vi "USRP_singlecarrierTDMUSRP1_withoutemu.vi"() -> ()   [LabVIEW 2021]
uses:
  <vilib>/addons/Modulation/Analog/controls/Complex Data Waveform.ctl
  <vilib>/Analysis/coordinate.llb/Angle Units.ctl
  <vilib>/Analysis/coordinate.llb/Angle Range (Degree).ctl
  <vilib>/Analysis/coordinate.llb/Wrap Angle (scalar).vi
  system stop.vi
  <vilib>/measure/matone.llb/Extract Single Tone Information 1 Chan (CDB).vi
  <instrlib>/niUSRP/niUSRP Fetch Rx Data (CDB Cluster).vi
  <instrlib>/niUSRP/niUSRP Write Tx Data (CDB Cluster).vi
  <vilib>/addons/Modulation/niAMT.lvlib
  <vilib>/measure/NI_MAPro.lvlib
  <vilib>/Analysis/NI_AAL_Angle.lvlib
panel:
  in  "Tab Control":T1(tab)
  in  "IQ rate Tx":dbl=400000.0 format="%#_6p"
  in  "Tx Gain":dbl format="%#_6f"
  in  "Tx IP":refnum<k15>="192.168.10.2"
  out "coerced IQ rate Tx":dbl=100000.0 format="%#_6p"
  out "coerced carrier frequency Tx":dbl=100000.0 format="%#_6p"
  in  "Rx IP":refnum<k15>="192.168.10.2"
  in  "Rx gain":dbl format="%#_6f"
  in  "Frequency":dbl=10000.0 format="%#_13g"
  in  "Duration":dbl=0.01 format="%#_13g"
  out "coerced IQ rate Rx":dbl=100000.0 format="%#_6p"
  out "coerced carrier frequency Rx":dbl=100000.0 format="%#_6p"
  in  "number of samples":i64=4000
  in  "carrier frequency":dbl=2400000000.0 format="%#_6p"
  in  "Phase in deg":dbl
  out "Waveform Graph":dbl[](graph)
  out "Boolean":bool
  out "detected frequency":dbl format="%.2p"
  out "detected Amplitude in dBm":dbl format="%.2p"
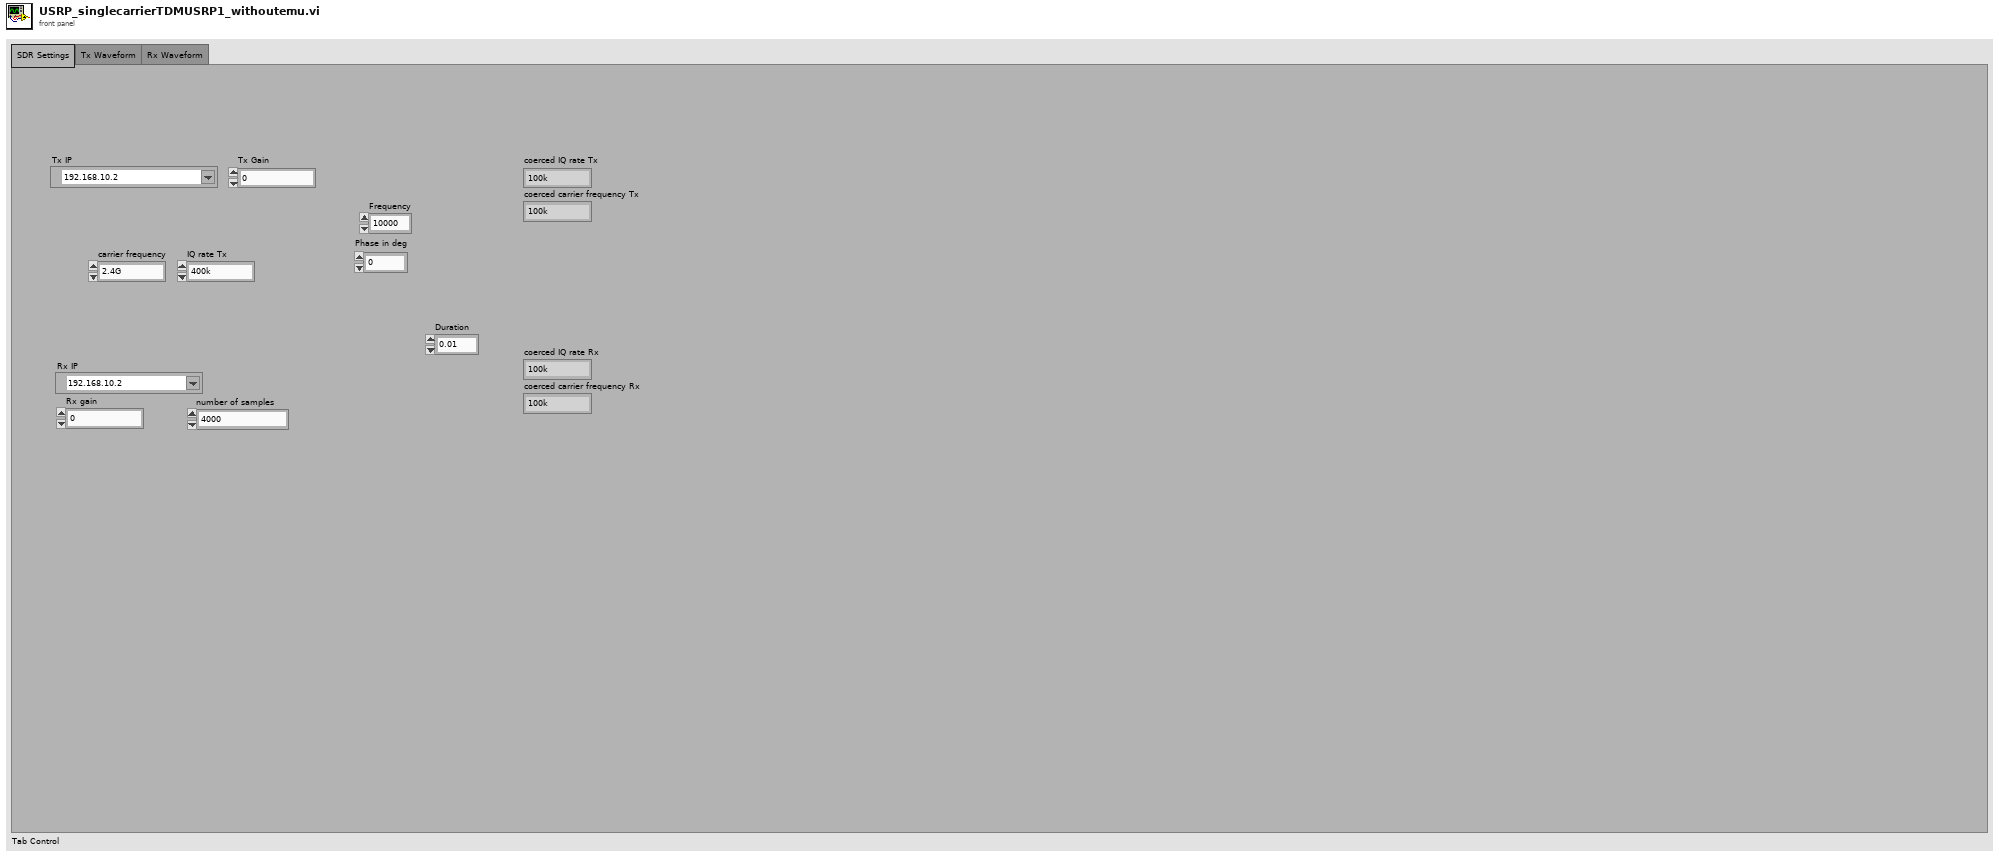
[diagram p1: front panel]
types:
  T1 = enum32{"SDR Settings", "Tx Waveform", "Rx Waveform"}
  T2 = typedef "niAMT.lvlib/Complex Data Waveform.ctl" = cluster{"t0":dbl, "dt":dbl, "Y":cdb[]}
  T3 = typedef "NI_AAL_Angle.lvlib/Angle Range (Degree).ctl" = u16
  T4 = typedef "NI_AAL_Angle.lvlib/Angle Units.ctl" = i32
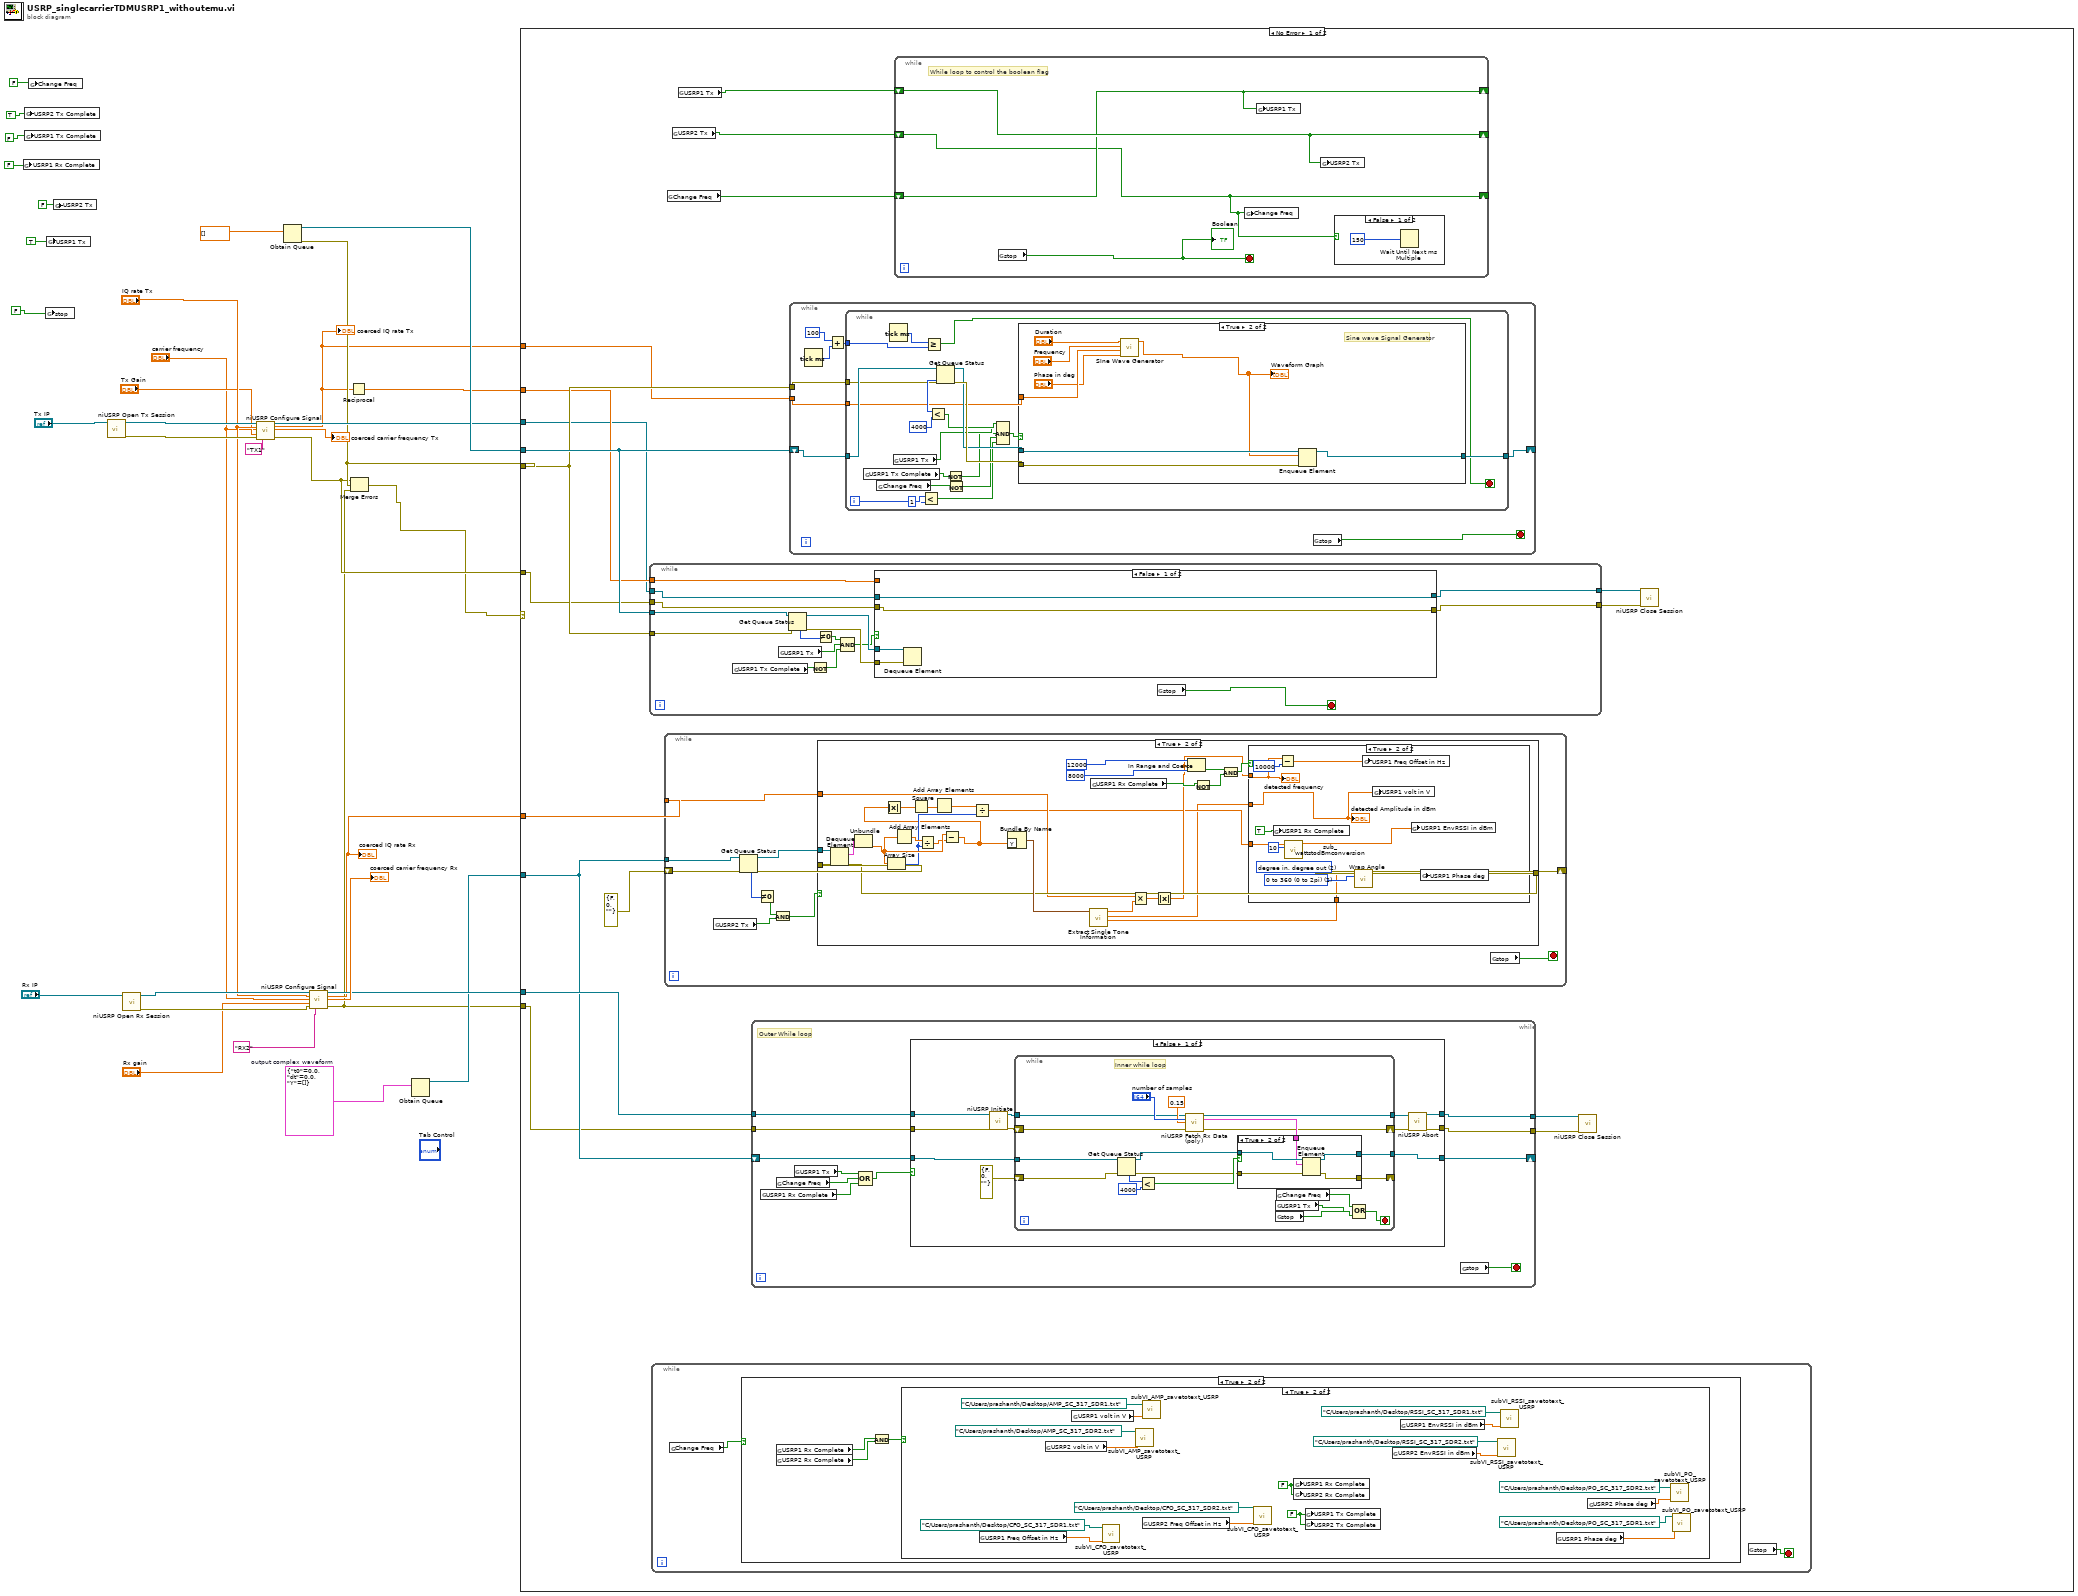
[diagram p0: block diagram]
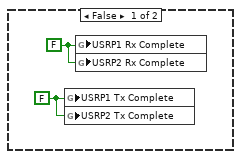
[diagram p3: hidden frame]
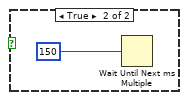
[diagram p4: hidden frame]
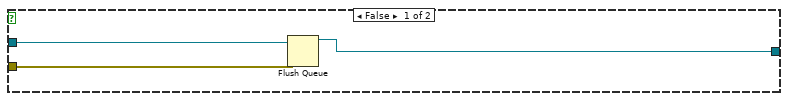
[diagram p5: hidden frame]
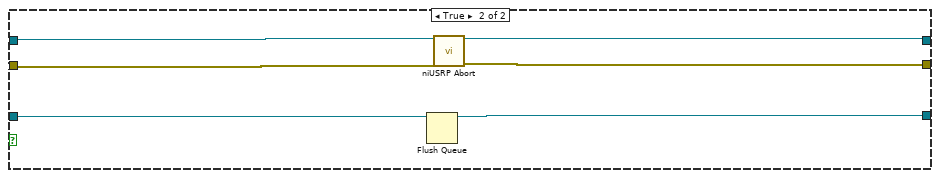
[diagram p7: hidden frame]
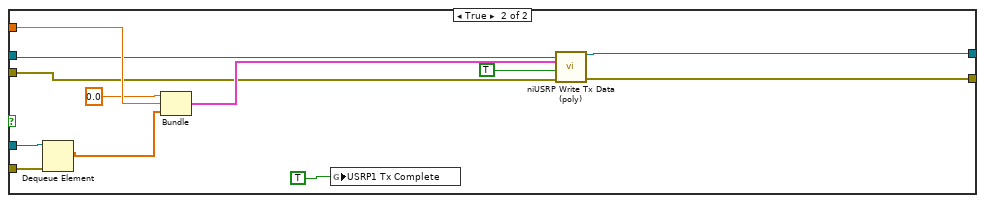
[diagram p10: hidden frame]
diagram:
  w8 = T2 {"t0"=0.0, "dt"=0.0, "Y"=[]}  # output complex waveform
  n1 = global write "system stop.vi" "USRP1 Rx Complete"(FALSE) -> ()
  n2 = global write "system stop.vi" "USRP2 Tx Complete"(TRUE) -> ()
  n3 = global write "system stop.vi" "USRP1 Tx Complete"(FALSE) -> ()
  n4 = global write "system stop.vi" "Change Freq"(FALSE) -> ()
  n5 = global write "system stop.vi" "stop"(FALSE) -> ()
  n6 = global write "system stop.vi" "USRP1 Tx"(TRUE) -> ()
  n7 = global write "system stop.vi" "USRP2 Tx"(FALSE) -> ()
  n8 = call <instrlib>:"niUSRP Open Tx Session.vi"("device names"="Tx IP") -> ("session handle out"=w33:refnum<k15>, "error out"=w32:errorcluster)  [unwired: 13 in]
  n9 = call <instrlib>:"niUSRP Open Rx Session.vi"("device names"="Rx IP") -> ("session handle out"=w30:refnum<k15>, "error out"=w29:errorcluster)  [unwired: 13 in]
  n10 = call <instrlib>:"niUSRP Configure Signal.vi"("session handle"=w33, "IQ rate"="IQ rate Tx", "carrier frequency"="carrier frequency", "gain"="Tx Gain", "error in (no error)"=w32, "active antenna"="TX1") -> ("session handle out"=w15:refnum<k15>, "coerced IQ rate"=w12:dbl, "coerced carrier frequency"=→"coerced carrier frequency Tx":dbl, "error out"=w11:errorcluster)  [unwired: 5 in, 1 out]
  "coerced IQ rate Tx" <- w12
  n11 = Obtain Queue(element data type=dbl[] []) -> (queue out=w16:refnum<queue>, error out=w13:errorcluster)  [unwired: 4 in, 1 out]
  n12 = call <instrlib>:"niUSRP Configure Signal.vi"("session handle"=w30, "IQ rate"="IQ rate Tx", "carrier frequency"="carrier frequency", "gain"="Rx gain", "error in (no error)"=w29, "active antenna"="RX2") -> ("session handle out"=w9:refnum<k15>, "coerced IQ rate"=w6:dbl, "coerced carrier frequency"=→"coerced carrier frequency Rx":dbl, "error out"=w5:errorcluster)  [unwired: 5 in, 1 out]
  "coerced IQ rate Rx" <- w6
  n13 = Reciprocal(x=w12) -> (1/x=w14:dbl)
  n14 = Merge Errors(w11, w13, w5) -> (w3:errorcluster)
  n15 = Obtain Queue(element data type=w8) -> (queue out=w7:refnum<queue>)  [unwired: 4 in, 2 out]
  n16 = case shown="No Error" w3 {
    tunnel: w13 -> [w51 _]
    tunnel: w16 -> [w52 _]
    tunnel: w15 -> [w49 _]
    tunnel: w14 -> [w50 _]
    tunnel: w12 -> [w48 _]
    tunnel: w11 -> [w47 _]
    tunnel: w9 -> [w45 _]
    tunnel: w7 -> [w44 _]
    tunnel: w6 -> [w43 _]
    tunnel: w5 -> [w42 _]
    frame No Error {
      n17 = while {
        tunnel: w52 -> [w244]
        tunnel: w51 -> [w241]
        tunnel: w50 -> [w240]
        tunnel: w49 -> [w237]
        tunnel: w47 -> [w236]
        tunnel: [w230] -> w38
        tunnel: [w229] -> w37
        stop <- w238 stop-if-true
        n18 = global read "system stop.vi" "USRP1 Tx Complete"() -> (w232:bool)
        n19 = global read "system stop.vi" "USRP1 Tx"() -> (w234:bool)
        n20 = Get Queue Status(queue=w244, error in (no error)=w241) -> (queue out=w243:refnum<queue>, error out=w242:errorcluster, # elements in queue=w239:i32)  [unwired: 1 in, 5 out]
        n21 = Not(x=w232) -> (.not. x?=w233:bool)
        n22 = Not Equal To 0?(x=w239) -> (x != 0?=w235:bool)
        n23 = Compound Arithmetic op=AND(w235, w234, w233) -> (w231:bool)
        n24 = case shown="False" w231 {
          tunnel: w243 -> [w246 w260]
          tunnel: w242 -> [w245 w259]
          tunnel: w240 -> [_ w258]
          tunnel: w237 -> [w248 w251]
          tunnel: w236 -> [w247 w250]
          tunnel: [w248 w254] -> w230
          tunnel: [w247 w252] -> w229
          frame False {
            n25 = Dequeue Element(queue=w246, error in (no error)=w245) -> ()  [unwired: 1 in, 4 out]
          }
          frame True {
            n26 = Dequeue Element(queue=w260, error in (no error)=w259) -> (element=w249:dbl[])  [unwired: 1 in, 3 out]
            n27 = Bundle(0.0, w258, w249) -> (w257:cluster{dbl, dbl, dbl[]})  [unwired: 1 in]
            n28 = global write "system stop.vi" "USRP1 Tx Complete"(TRUE) -> ()
            n29 = call-poly <instrlib>:"niUSRP Write Tx Data (poly).vi"("session handle"=w251, "data"=w257, "end of data?"=TRUE, "error in (no error)"=w250) -> ("session handle out"=w254:refnum<k15>, "error out"=w252:errorcluster)  [unwired: 10 in]
          }
        }
        n30 = global read "system stop.vi" "stop"() -> (w238:bool)
      }
      n31 = while {
        stop <- w53 stop-if-true
        n32 = global read "system stop.vi" "Change Freq"() -> (w54:bool)
        n33 = case shown="True" w54 {
          frame False {
          }
          frame True {
            n34 = global read "system stop.vi" "USRP1 Rx Complete"() -> (w57:bool)
            n35 = global read "system stop.vi" "USRP2 Rx Complete"() -> (w56:bool)
            n36 = And(x=w57, y=w56) -> (x .and. y?=w55:bool)
            n37 = case shown="True" w55 {
              frame False {
                w59 = FALSE
                w58 = FALSE
                n38 = global write "system stop.vi" "USRP1 Tx Complete"(w59) -> ()
                n39 = global write "system stop.vi" "USRP2 Tx Complete"(w59) -> ()
                n40 = global write "system stop.vi" "USRP1 Rx Complete"(w58) -> ()
                n41 = global write "system stop.vi" "USRP2 Rx Complete"(w58) -> ()
              }
              frame True {
                w77 = FALSE
                w76 = FALSE
                n42 = global read "system stop.vi" "USRP1 Freq Offset in Hz"() -> (w70:dbl)
                n43 = global read "system stop.vi" "USRP2 volt in V"() -> (w73:dbl)
                n44 = global read "system stop.vi" "USRP1 volt in V"() -> (w74:dbl)
                n45 = call "subVI_CFO_savetotext_USRP.vi"("RSSI"=w70, "file path (dialog if empty)"=path "C:/Users/prashanth/Desktop/CFO_SC_317_SDR1.txt") -> ()  [unwired: 10 in]
                n46 = call "subVI_AMP_savetotext_USRP.vi"("RSSI"=w73, "file path (dialog if empty)"=path "C:/Users/prashanth/Desktop/AMP_SC_317_SDR2.txt") -> ()  [unwired: 10 in]
                n47 = call "subVI_AMP_savetotext_USRP.vi"("RSSI"=w74, "file path (dialog if empty)"=path "C:/Users/prashanth/Desktop/AMP_SC_317_SDR1.txt") -> ()  [unwired: 10 in]
                n48 = global read "system stop.vi" "USRP2 Freq Offset in Hz"() -> (w68:dbl)
                n49 = call "subVI_CFO_savetotext_USRP.vi"("RSSI"=w68, "file path (dialog if empty)"=path "C:/Users/prashanth/Desktop/CFO_SC_317_SDR2.txt") -> ()  [unwired: 10 in]
                n50 = global write "system stop.vi" "USRP1 Rx Complete"(w76) -> ()
                n51 = global write "system stop.vi" "USRP2 Rx Complete"(w76) -> ()
                n52 = global write "system stop.vi" "USRP1 Tx Complete"(w77) -> ()
                n53 = global write "system stop.vi" "USRP2 Tx Complete"(w77) -> ()
                n54 = global read "system stop.vi" "USRP2 EnvRSSI in dBm"() -> (w66:dbl)
                n55 = global read "system stop.vi" "USRP1 EnvRSSI in dBm"() -> (w64:dbl)
                n56 = call "subVI_RSSI_savetotext_USRP.vi"("RSSI"=w66, "file path (dialog if empty)"=path "C:/Users/prashanth/Desktop/RSSI_SC_317_SDR2.txt") -> ()  [unwired: 10 in]
                n57 = call "subVI_RSSI_savetotext_USRP.vi"("RSSI"=w64, "file path (dialog if empty)"=path "C:/Users/prashanth/Desktop/RSSI_SC_317_SDR1.txt") -> ()  [unwired: 10 in]
                n58 = global read "system stop.vi" "USRP1 Phase deg"() -> (w62:dbl)
                n59 = global read "system stop.vi" "USRP2 Phase deg"() -> (w60:dbl)
                n60 = call "subVI_PO_savetotext_USRP.vi"("RSSI"=w60, "file path (dialog if empty)"=path "C:/Users/prashanth/Desktop/PO_SC_317_SDR2.txt") -> ()  [unwired: 10 in]
                n61 = call "subVI_PO_savetotext_USRP.vi"("RSSI"=w62, "file path (dialog if empty)"=path "C:/Users/prashanth/Desktop/PO_SC_317_SDR1.txt") -> ()  [unwired: 10 in]
              }
            }
          }
        }
        n62 = global read "system stop.vi" "stop"() -> (w53:bool)
      }
      n63 = while {
        tunnel: w44 -> [w186]
        shift-right: [w184] -> _
        shift-left: errorcluster {"status"=FALSE, "code"=0, "source"=""} ("error in (no error)") -> [w185]
        tunnel: w43 -> [w183]
        stop <- w182 stop-if-true
        n64 = global read "system stop.vi" "USRP2 Tx"() -> (w181:bool)
        n65 = Get Queue Status(queue=w186, error in (no error)=w185) -> (queue out=w188:refnum<queue>, error out=w187:errorcluster, # elements in queue=w189:i32)  [unwired: 1 in, 5 out]
        n66 = Not Equal To 0?(x=w189) -> (x != 0?=w180:bool)
        n67 = And(x=w180, y=w181) -> (x .and. y?=w179:bool)
        n68 = case shown="True" w179 {
          tunnel: w188 -> [_ w216]
          tunnel: w187 -> [w190 w215]
          tunnel: [w190 w205] -> w184
          tunnel: w183 -> [_ w203]
          frame False {
          }
          frame True {
            n69 = Dequeue Element(queue=w216, error in (no error)=w215) -> (element=w214:T2, error out=w205:errorcluster)  [unwired: 1 in, 2 out]
            n70 = Unbundle(w214) -> ("Y"=w200:cdb[])  [unwired: 2 out]
            n71 = Array Size(array=w200) -> (size(s)=w197:i32)
            n72 = Add Array Elements(numeric array=w200) -> (sum=w213:cdb)
            n73 = Divide(x=w213, y=w197) -> (x/y=w198:cdb)
            n74 = Subtract(x=w200, y=w198) -> (x-y=w192:cdb[])
            n75 = Absolute Value(x=w192) -> (abs(x)=w199:dbl[])
            n76 = Square(x=w199) -> (x^2=w196:dbl[])
            n77 = Add Array Elements(numeric array=w196) -> (sum=w195:dbl)
            n78 = Divide(x=w195, y=w197) -> (x/y=w194:dbl)
            n79 = Bundle By Name("Y"=w192) -> (w206:waveform(cdb))  [unwired: 1 in]
            n80 = call-poly <vilib>:"Extract Single Tone Information.vi"("time signal in"=w206) -> ("detected phase (deg)"=w193:dbl, "detected amplitude"=w191:dbl, "detected frequency"=w204:dbl)  [unwired: 5 in, 3 out]
            n81 = global read "system stop.vi" "USRP1 Rx Complete"() -> (w208:bool)
            n82 = Multiply(x=w203, y=w204) -> (x*y=w202:dbl)
            n83 = Absolute Value(x=w202) -> (abs(x)=w201:dbl)
            n84 = In Range and Coerce(upper limit=12000, x=w201, lower limit=8000) -> (In Range?=w209:bool)  [unwired: 1 out]
            n85 = Not(x=w208) -> (.not. x?=w207:bool)
            n86 = And(x=w209, y=w207) -> (x .and. y?=w210:bool)
            n87 = case shown="True" w210 {
              tunnel: w201 -> [_ w227]
              tunnel: w191 -> [_ w217]
              tunnel: w194 -> [_ w224]
              tunnel: w193 -> [_ w219]
              frame False {
              }
              frame True {
                w221 = T3 2 items=["none", "-180 to 180 (-pi to pi)", "0 to 360 (0 to 2pi)"] ("angle range")
                w222 = T4 2 items=["radian in, radian out", "radian in, degree out", "degree in, degree out", "degree in, radian out"] ("angle units")
                n88 = global write "system stop.vi" "USRP1 Rx Complete"(TRUE) -> ()
                n89 = Subtract(x=w227, y=10000) -> (x-y=w225:dbl)
                n90 = call "sub_wattstodBmconversion.vi"("Amp or Power"=10, "detected amplitude"=w224) -> ("Numeric"=w223:dbl)  [unwired: 9 in]
                n91 = call-poly <vilib>:"Wrap Angle.vi"("angle units"=w222, "angle range"=w221, "angle in"=w219) -> ("angle out"=w220:dbl)  [unwired: 7 in, 1 out]
                n92 = global write "system stop.vi" "USRP1 Freq Offset in Hz"(w225) -> ()
                n93 = global write "system stop.vi" "USRP1 volt in V"(w217) -> ()
                n94 = global write "system stop.vi" "USRP1 EnvRSSI in dBm"(w223) -> ()
                n95 = global write "system stop.vi" "USRP1 Phase deg"(w220) -> ()
                "detected frequency" <- w227
                "detected Amplitude in dBm" <- w217
              }
            }
          }
        }
        n96 = global read "system stop.vi" "stop"() -> (w182:bool)
      }
      n97 = global read "system stop.vi" "Change Freq"() -> (w40:bool)
      n98 = global read "system stop.vi" "USRP2 Tx"() -> (w39:bool)
      n99 = global read "system stop.vi" "USRP1 Tx"() -> (w41:bool)
      n100 = while {
        shift-right: [w130] -> _
        shift-left: w44 -> [w134]
        tunnel: w45 -> [w132]
        tunnel: w42 -> [w131]
        tunnel: [w125] -> w36
        tunnel: [w124] -> w35
        stop <- w133 stop-if-true
        # "Outer While loop"
        n101 = global read "system stop.vi" "USRP1 Rx Complete"() -> (w128:bool)
        n102 = global read "system stop.vi" "Change Freq"() -> (w126:bool)
        n103 = global read "system stop.vi" "USRP1 Tx"() -> (w127:bool)
        n104 = Compound Arithmetic op=OR(w127, w126, w128) -> (w129:bool)
        n105 = case shown="False" w129 {
          tunnel: w132 -> [w137 w178]
          tunnel: w134 -> [w145 w174]
          tunnel: w131 -> [w136 w176]
          tunnel: [w140 w177] -> w125
          tunnel: [w139 w175] -> w124
          tunnel: [w135 w173] -> w130
          frame False {
            n106 = call <instrlib>:"niUSRP Initiate.vi"("session handle"=w137, "error in (no error)"=w136) -> ("session handle out"=w143:refnum<k15>, "error out"=w142:errorcluster)  [unwired: 12 in]
            n107 = while {
              tunnel: w145 -> [w165]
              shift-right: [w149] -> w138
              shift-left: w142 -> [w151]
              shift-right: [w164] -> _
              shift-left: errorcluster {"status"=FALSE, "code"=0, "source"=""} ("error in (no error)") -> [w163]
              tunnel: w143 -> [w152]
              tunnel: [w150] -> w141
              tunnel: [w146] -> w135
              stop <- w155 stop-if-true
              # "Inner while loop"
              n108 = Get Queue Status(queue=w165, error in (no error)=w163) -> (queue out=w158:refnum<queue>, error out=w159:errorcluster, # elements in queue=w162:i32)  [unwired: 1 in, 5 out]
              n109 = Less?(x=w162, y=4000) -> (x < y?=w160:bool)
              n110 = call-poly <instrlib>:"niUSRP Fetch Rx Data (poly).vi"("session handle"=w152, "number of samples"="number of samples", "timeout"=0.15, "error in (no error)"=w151) -> ("session handle out"=w150:refnum<k15>, "data"=w156:cluster{"t0":dbl, "dt":dbl, "Y":cdb[]}, "error out"=w149:errorcluster)  [unwired: 8 in, 1 out]
              n111 = case shown="True" w160 {
                tunnel: w159 -> [w167 w172]
                tunnel: w158 -> [w166 w171]
                tunnel: w156 -> [_ w170]
                tunnel: [w167 w169] -> w164
                tunnel: [w166 w168] -> w146
                frame False {
                }
                frame True {
                  n112 = Enqueue Element(queue=w171, element=w170, error in (no error)=w172) -> (queue out=w168:refnum<queue>, error out=w169:errorcluster)  [unwired: 1 in, 1 out]
                }
              }
              n113 = global read "system stop.vi" "USRP1 Tx"() -> (w148:bool)
              n114 = global read "system stop.vi" "stop"() -> (w154:bool)
              n115 = global read "system stop.vi" "Change Freq"() -> (w147:bool)
              n116 = Compound Arithmetic op=OR(w147, w148, w154) -> (w155:bool)
            }
            n117 = call <instrlib>:"niUSRP Abort.vi"("session handle"=w141, "error in (no error)"=w138) -> ("session handle out"=w140:refnum<k15>, "error out"=w139:errorcluster)  [unwired: 12 in]
          }
          frame True {
            n118 = Flush Queue(queue=w174) -> (queue out=w173:refnum<queue>)  [unwired: 1 in, 2 out]
            n119 = call <instrlib>:"niUSRP Abort.vi"("session handle"=w178, "error in (no error)"=w176) -> ("session handle out"=w177:refnum<k15>, "error out"=w175:errorcluster)  [unwired: 12 in]
          }
        }
        n120 = global read "system stop.vi" "stop"() -> (w133:bool)
      }
      n121 = while {
        tunnel: w51 -> [w90]
        tunnel: w48 -> [w89]
        shift-right: [w84] -> _
        shift-left: w52 -> [w91]
        stop <- w85 stop-if-true
        n122 = Tick Count (ms)() -> (millisecond timer value=w87:u32)
        n123 = Add(x=100, y=w87) -> (x+y=w86:u32)
        n124 = while {
          tunnel: w90 -> [w107]
          tunnel: w89 -> [w106]
          tunnel: w86 -> [w101]
          tunnel: w91 -> [w108]
          tunnel: [w99] -> w84
          i -> [w94]
          stop <- w96 stop-if-true
          n125 = global read "system stop.vi" "USRP1 Tx Complete"() -> (w98:bool)
          n126 = global read "system stop.vi" "Change Freq"() -> (w97:bool)
          n127 = Tick Count (ms)() -> (millisecond timer value=w102:u32)
          n128 = global read "system stop.vi" "USRP1 Tx"() -> (w104:bool)
          n129 = Less?(x=w94, y=1) -> (x < y?=w92:bool)
          n130 = Greater Or Equal?(x=w102, y=w101) -> (x >= y?=w96:bool)
          n131 = Get Queue Status(queue=w108, error in (no error)=w107) -> (queue out=w109:refnum<queue>, error out=w110:errorcluster, # elements in queue=w112:i32)  [unwired: 1 in, 5 out]
          n132 = Less?(x=w112, y=4000) -> (x < y?=w105:bool)
          n133 = Not(x=w98) -> (.not. x?=w100:bool)
          n134 = Not(x=w97) -> (.not. x?=w95:bool)
          n135 = Compound Arithmetic op=AND(w105, w104, w100, w95, w92) -> (w103:bool)
          n136 = case shown="True" w103 {
            tunnel: w110 -> [w114 w123]
            tunnel: w109 -> [w115 w122]
            tunnel: w106 -> [_ w118]
            tunnel: [w113 w120] -> w99
            frame False {
              n137 = Flush Queue(queue=w115, error in (no error)=w114) -> (queue out=w113:refnum<queue>)  [unwired: 2 out]
            }
            frame True {
              # "Sine wave Signal Generator"
              n138 = call "SIne Wave Generator.vi"("Phase in deg"="Phase in deg", "Sampling rate"=w118, "Frequency"="Frequency", "Duration"="Duration") -> ("Array"=w116:dbl[])  [unwired: 6 in, 1 out]
              "Waveform Graph" <- w116
              n139 = Enqueue Element(queue=w122, element=w116, error in (no error)=w123) -> (queue out=w120:refnum<queue>)  [unwired: 1 in, 2 out]
            }
          }
        }
        n140 = global read "system stop.vi" "stop"() -> (w85:bool)
      }
      n141 = while {
        shift-right: [w79] -> _
        shift-left: w41 -> [w81]
        shift-right: [w81] -> _
        shift-left: w39 -> [w78]
        shift-right: [w78] -> _
        shift-left: w40 -> [w79]
        stop <- w80 stop-if-true
        # "While loop to control the boolean flag"
        n142 = global read "system stop.vi" "stop"() -> (w80:bool)
        "Boolean" <- w80
        n143 = global write "system stop.vi" "Change Freq"(w78) -> ()
        n144 = global write "system stop.vi" "USRP1 Tx"(w79) -> ()
        n145 = global write "system stop.vi" "USRP2 Tx"(w81) -> ()
        n146 = case shown="False" w78 {
          frame False {
            n147 = Wait Until Next ms Multiple(millisecond multiple=150) -> ()  [unwired: 1 out]
          }
          frame True {
            n148 = Wait Until Next ms Multiple(millisecond multiple=150) -> ()  [unwired: 1 out]
          }
        }
      }
      n149 = call <instrlib>:"niUSRP Close Session.vi"("session handle"=w36, "error in (no error)"=w35) -> ()  [unwired: 13 in, 1 out]
      n150 = call <instrlib>:"niUSRP Close Session.vi"("session handle"=w38, "error in (no error)"=w37) -> ()  [unwired: 13 in, 1 out]
    }
    frame Error {
    }
  }
